vi "IsIdle.vi"(8 "Error In":errorcluster, 11 "Keithley 7001 In":refnum<visa-resource-name>) -> (0 "Error Out":errorcluster, 2 "Idle?":bool, 3 "Keithley 7001 Out":refnum<visa-resource-name>)   [LabVIEW 2012, in "Keithley-7001.lvlib"]
uses:
  Keithley-7001.lvlib
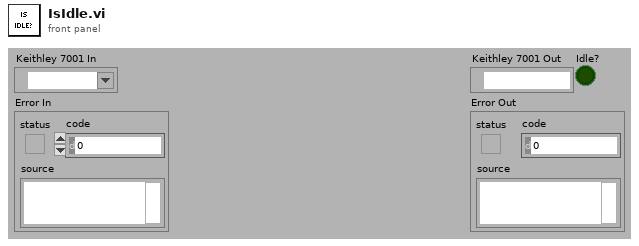
[diagram p1: front panel]
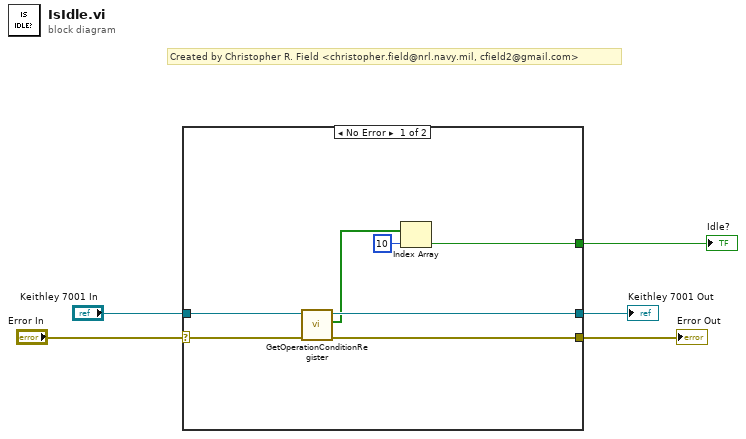
[diagram p0: block diagram]
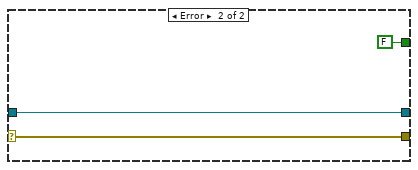
[diagram p2: hidden frame]
diagram:
  # "Created by Christopher R. Field <christopher.field@nrl.navy.mil, cfield2@gmail.com>"
  n1 = case shown="No Error" "Error In" {
    selector: "Error In" -> [w6 w15]
    tunnel: "Keithley 7001 In" -> [w12 w14]
    tunnel: [w11 w14] -> w4
    tunnel: [w10 w15] -> w3
    tunnel: [w7 FALSE] -> w2
    frame No Error {
      n2 = call "GetOperationConditionRegister.vi"("Error In"=w6, "Keithley 7001 In"=w12) -> ("Error Out"=w10:errorcluster, "Operation Condition Register"=w9:bool[], "Keithley 7001 Out"=w11:refnum<visa-resource-name>)  [unwired: 7 in]
      n3 = Index Array(array=w9, index=10) -> (element=w7:bool)
    }
    frame Error {
    }
  }
  "Keithley 7001 Out" <- w4
  "Error Out" <- w3
  "Idle?" <- w2
